vi "ParseArguments.vi"(8 "error in (no error)":errorcluster, 9 "Inputs":string[](array[string]), 11 "SecureRunVI in":refnum<class "SecureRunVI.lvclass">) -> (0 "error out":errorcluster, 3 "SecureRunVI out":refnum<class "SecureRunVI.lvclass">)   [LabVIEW 2014, in "SecureRunVI.lvclass"]
doc: "Parses command line arguments passed through LabVIEWCLI."
uses:
  SecureRunVI.lvclass
  SecureRunVI.lvclass/SecureRunVI.ctl
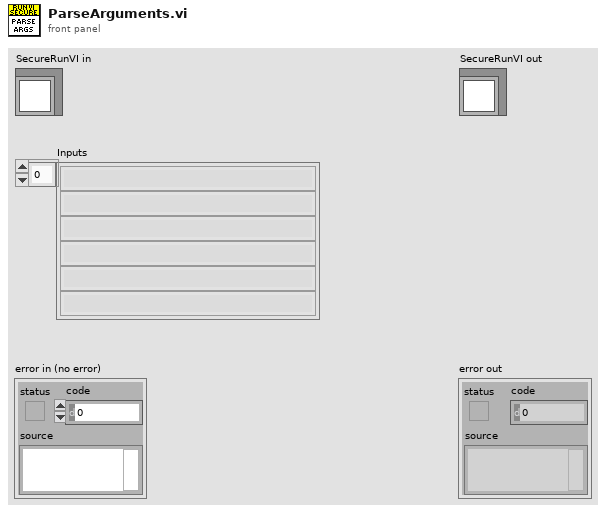
[diagram p1: front panel]
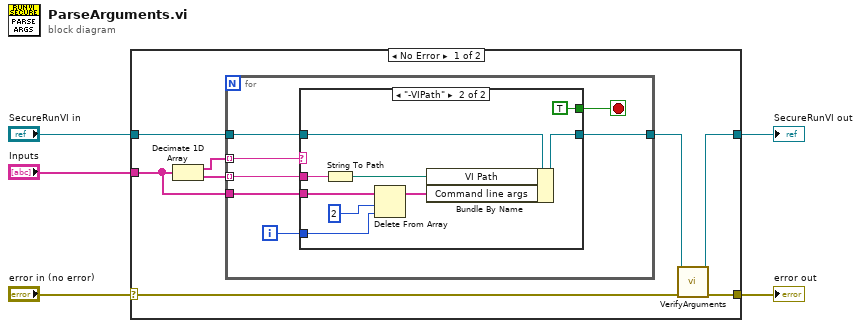
[diagram p0: block diagram]
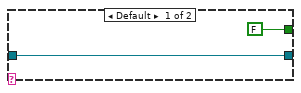
[diagram p2: hidden frame]
diagram:
  n1 = case shown="No Error" "error in (no error)" {
    selector: "error in (no error)" -> [w9 w33]
    tunnel: [w8 w33] -> w4
    tunnel: [w7 w32] -> w2
    tunnel: "SecureRunVI in" -> [w11 w32]
    tunnel: "Inputs" -> [w10 _]
    frame No Error {
      n2 = Decimate 1D Array(w10) -> (w12:string[], w13:string[])
      n3 = for {
        tunnel: w12 -> [w20] mode=indexing
        tunnel: w11 -> [w19]
        tunnel: [w17] -> w6
        tunnel: w13 -> [w16] mode=indexing
        tunnel: w10 -> [w14]
        i -> [w15]
        stop <- w18 stop-if-true
        n4 = case shown="\"-VIPath\"" w20 {
          tunnel: w19 -> [w21 w30]
          tunnel: [FALSE TRUE] -> w18
          tunnel: [w21 w29] -> w17
          tunnel: w16 -> [_ w27]
          tunnel: w15 -> [_ w26]
          tunnel: w14 -> [_ w24]
          frame Default {
          }
          frame "-VIPath" {
            n5 = String To Path(string=w27) -> (path=w28:path)
            n6 = Delete From Array(array=w24, length=2, index=w26) -> (array with subset deleted=w23:string[])  [unwired: 1 out]
            n7 = Bundle By Name(cluster=w30, "VI Path"=w28, "Command line args"=w23) -> (w29:refnum<class "SecureRunVI.lvclass">)
          }
        }
      }
      n8 = call "VerifyArguments.vi"("error in (no error)"=w9, "SecureRunVI in"=w6) -> ("error out"=w8:errorcluster, "SecureRunVI out"=w7:refnum<class "SecureRunVI.lvclass">)  [unwired: 8 in]
    }
    frame Error {
    }
  }
  "error out" <- w4
  "SecureRunVI out" <- w2
